vi "DMM Driver Test.vi"() -> ()   [LabVIEW 2011]
uses:
  DMM Driver Ref.ctl
  DMM Command.ctl
  tests/DC Attenuation/TypeDefs/DCA Stimulus Parameters.ctl
  DMM Measurement.ctl
panel:
  in  "Tab Control":enum32{"Stimulus", "Measurements"}(tab)=enum."Measurements"
  out "Get Stimulus":T1
  in  "get stimulus":bool
  in  "set stimulus":bool
  in  "Set Stimulus":T1
  out "DMM Measurement":T2 caption="This reading is allways in the base units\ni.e. V, A, Ohms, Hz, Sec, etc." format="%#_10f"
  in  "measure":bool
  in  "preset":bool
  in  "config":bool
  in  "init":bool
  in  "VNA Drivers":u16(ring) items=["Agilent DMM", "Summitek DMM"]
  in  "load":bool
  in  "stop":bool
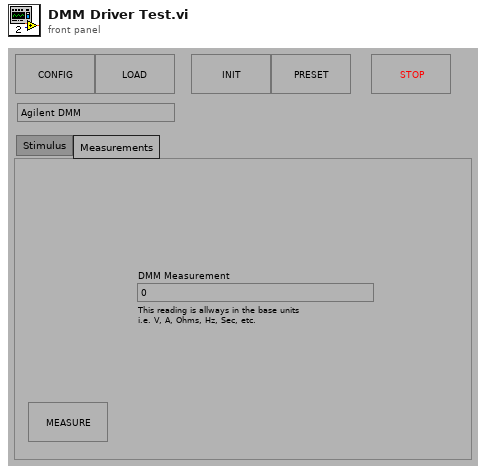
[diagram p1: front panel]
types:
  T1 = typedef "DCA Stimulus Parameters.ctl" = cluster{"Use Instrument":bool, "Normalize":bool, "Blank Screen":bool, "Measurement Type":enum16{"Voltage DC", "Voltage DC Ratio", "Voltage AC", "Current DC", "Current AC", "Resistance", "Fresistance", "Frequency", "Period", "Continuity", "Diode"}, "Range":enum16{"Auto", "Minimum", "Maximum", "100", "1,000", "10,000", "100,000", "1,000,000", "10,000,000", "100,000,000"}, "Resolution":enum16{"Auto", "4 1/2", "5 1/2", "6 1/2"}}
  T2 = typedef "DMM Measurement.ctl" = dbl
  T3 = typedef "DMM Driver Ref.ctl" = refnum<vi>
  T4 = typedef "DMM Command.ctl" = enum16{"LOAD", "INITIALIZE", "PRESET", "GET STIMULUS", "SET STIMULUS", "MEASURE", "RELEASE", "UNLOAD", "GET CALIBRATION", "CALIBRATE"}
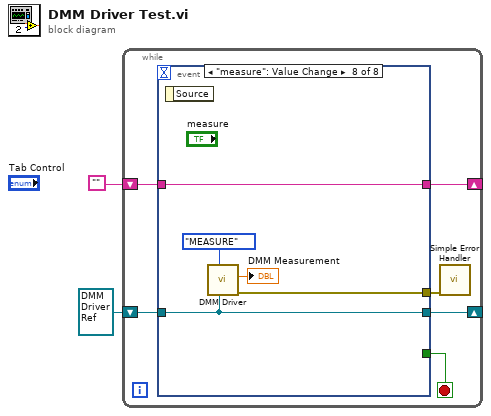
[diagram p0: block diagram]
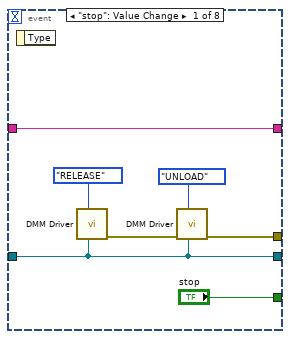
[diagram p2: hidden frame]
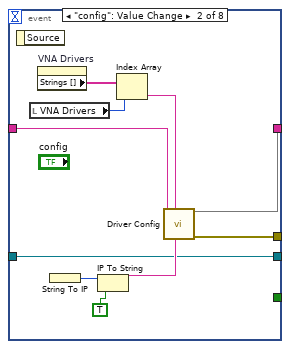
[diagram p3: hidden frame]
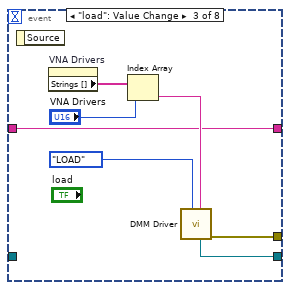
[diagram p4: hidden frame]
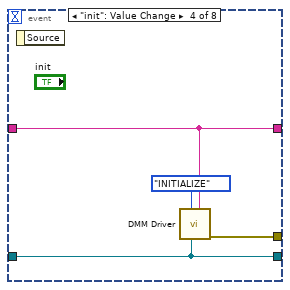
[diagram p5: hidden frame]
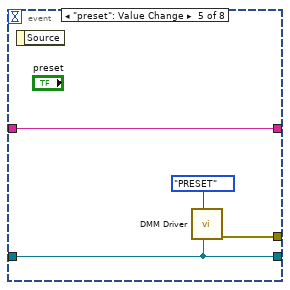
[diagram p6: hidden frame]
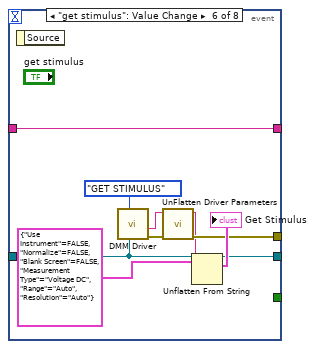
[diagram p7: hidden frame]
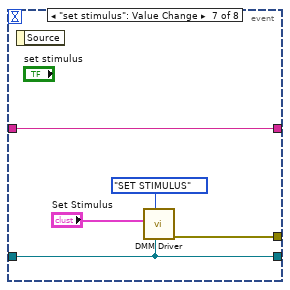
[diagram p8: hidden frame]
diagram:
  n1 = while {
    shift-right: [w6] -> _
    shift-left: "" -> [w5]
    shift-right: [w3] -> _
    shift-left: T3 refnum ("Driver Ref") -> [w4]
    stop <- w8 stop-if-true
    n2 = event shown="[7] \"measure\": Value Change" {
      selector: _ -> [_ _ _ _ _ _ _ _]
      dyn-events: _ -> [_ _ _ _ _ _ _ _]
      timeout: _ -> [_ _ _ _ _ _ _ _]
      tunnel: ["stop" _ _ _ _ _ _ _] -> w8
      tunnel: [w11 w25 w28 w36 w40 w43 w52 w57] -> w7
      tunnel: [w14 w24 w27 w33 w39 w49 w54 w59] -> w6
      tunnel: w5 -> [w14 w23 w27 w33 w39 w49 w54 w59]
      tunnel: w4 -> [w9 w16 _ w34 w37 w45 w50 w56]
      tunnel: [w9 w16 w26 w34 w37 w45 w50 w56] -> w3
      event "stop": Value Change {
        n3 = event-data() -> ()  [unwired: 1 in, 1 out]
        n4 = call "DMM Driver.vi"("Drv Refnum"=w9, "DMM Command"=DMM_Command."RELEASE" ("VNA Command")) -> ("error out"=w12:errorcluster)  [unwired: 6 in, 3 out]
        n5 = call "DMM Driver.vi"("Drv Refnum"=w9, "DMM Command"=DMM_Command."UNLOAD" ("VNA Command"), "error in (no error)"=w12) -> ("error out"=w11:errorcluster)  [unwired: 5 in, 3 out]
      }
      event "config": Value Change {
        n6 = event-data() -> ()  [unwired: 1 in, 1 out]
        n7 = local read "VNA Drivers"() -> (w19:u16)
        n8 = property on="VNA Drivers" class="Ring (strict)"() -> ("Strings []"=w18:string[])  [unwired: 2 in, 2 out]
        n9 = String To IP() -> (0:w22:u32)  [unwired: 1 in]
        n10 = IP To String(1:TRUE, 2:w22) -> (0:w21:string)
        n11 = Index Array(array=w18, index=w19) -> (element=w17:string)
        n12 = call "Driver Config.vi"("CalDue"=w21, "DriverType (\"\")"=w17, "TestStation Client (\"\")"=w23) -> ("error out"=w25:errorcluster, 3:w24)  [unwired: 4 in, 3 out]
      }
      event "load": Value Change {
        n13 = event-data() -> ()  [unwired: 1 in, 1 out]
        n14 = property on="VNA Drivers" class="Ring (strict)"() -> ("Strings []"=w31:string[])  [unwired: 2 in, 2 out]
        n15 = Index Array(array=w31, index="VNA Drivers") -> (element=w29:string)
        n16 = call "DMM Driver.vi"("DMM Configuration (\"\")"=w29, "DMM Command"=DMM_Command."LOAD" ("VNA Command")) -> ("error out"=w28:errorcluster, "dup Drv Refnum"=w26:T3)  [unwired: 6 in, 2 out]
      }
      event "init": Value Change {
        n17 = event-data() -> ()  [unwired: 1 in, 1 out]
        n18 = call "DMM Driver.vi"("DMM Configuration (\"\")"=w33, "Drv Refnum"=w34, "DMM Command"=DMM_Command."INITIALIZE" ("VNA Command")) -> ("error out"=w36:errorcluster)  [unwired: 5 in, 3 out]
      }
      event "preset": Value Change {
        n19 = event-data() -> ()  [unwired: 1 in, 1 out]
        n20 = call "DMM Driver.vi"("Drv Refnum"=w37, "DMM Command"=DMM_Command."PRESET" ("VNA Command")) -> ("error out"=w40:errorcluster)  [unwired: 6 in, 3 out]
      }
      event "get stimulus": Value Change {
        n21 = event-data() -> ()  [unwired: 1 in, 1 out]
        n22 = call "DMM Driver.vi"("Drv Refnum"=w45, "DMM Command"=DMM_Command."GET STIMULUS" ("VNA Command")) -> ("error out"=w44:errorcluster, "DMM Flat Output"=w42:string)  [unwired: 6 in, 2 out]
        n23 = call "UnFlatten Driver Parameters.vi"("error in (no error)"=w44, "Flattened Driver Parameters with Version (\"\")"=w42) -> ("error out"=w43:errorcluster, "Flat Driver Parameters"=w41:string)  [unwired: 3 in, 1 out]
        n24 = Unflatten From String(type=T1 {"Use Instrument"=FALSE, "Normalize"=FALSE, "Blank Screen"=FALSE, "Measurement Type"=enum."Voltage DC", "Range"=enum."Auto", "Resolution"=enum."Auto"} ("Get Stimulus"), binary string=w41) -> (value=→"Get Stimulus":T1)  [unwired: 3 in, 2 out]
      }
      event "set stimulus": Value Change {
        n25 = event-data() -> ()  [unwired: 1 in, 1 out]
        n26 = call "DMM Driver.vi"("Drv Refnum"=w50, "DMM Command"=DMM_Command."SET STIMULUS" ("VNA Command"), "DMM Stimulus"="Set Stimulus") -> ("error out"=w52:errorcluster)  [unwired: 5 in, 3 out]
      }
      event "measure": Value Change {
        n27 = event-data() -> ()  [unwired: 1 in, 1 out]
        n28 = call "DMM Driver.vi"("Drv Refnum"=w56, "DMM Command"=DMM_Command."MEASURE" ("VNA Command")) -> ("error out"=w57:errorcluster, "DMM Measurement"=→"DMM Measurement":T2)  [unwired: 6 in, 2 out]
      }
    }
    n29 = call <vilib>:"Simple Error Handler.vi"("error in (no error)"=w7) -> ()  [unwired: 4 in, 5 out]
  }
